vi "Diagnostic Cycle.vi"(8 "error in (no error)":errorcluster, 11 "MSX-E3711 in":refnum<class "MSX-E3711.lvclass">) -> (0 "error out":errorcluster, 3 "MSX-E3711 out":refnum<class "MSX-E3711.lvclass">)   [LabVIEW 2014, in "MSX-E3711.lvlib" / "MSX-E3711.lvclass"]
uses:
  MSX-E3711.lvclass
  MSX-E3711.lvclass/MSX-E3711.ctl
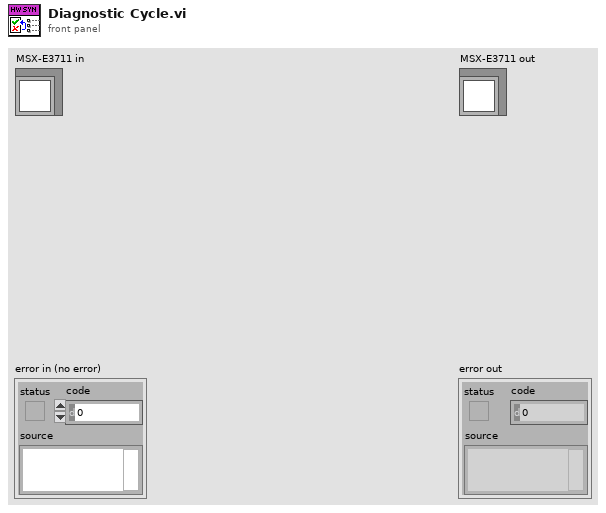
[diagram p1: front panel]
types:
  T1 = typedef "DriverMasterSync.lvlibp/WINFAS 2 Data Queue.lvlib/Acquisition Data 1 Sample Cluster.ctl" = cluster{"TDX":sgl[], "Encoder":sgl}
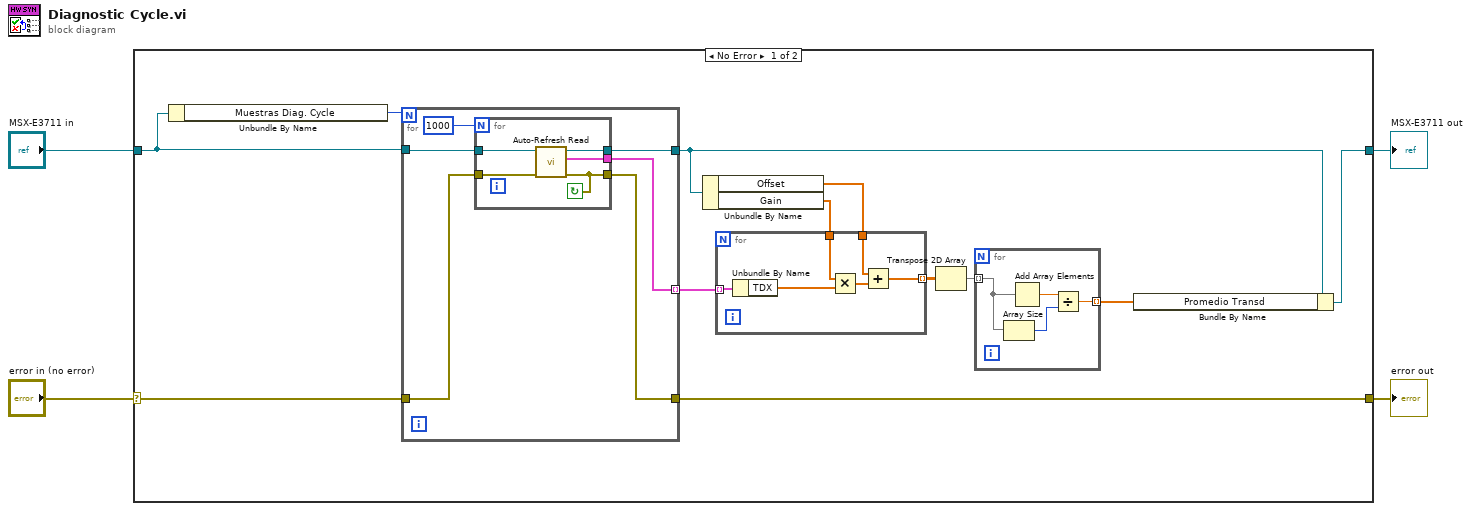
[diagram p0: block diagram]
diagram:
  n1 = case shown="No Error" "error in (no error)" {
    selector: "error in (no error)" -> [w8 w39]
    tunnel: [w5 w39] -> w3
    tunnel: [w6 w38] -> w1
    tunnel: "MSX-E3711 in" -> [w7 w38]
    frame No Error {
      n2 = Unbundle By Name(w7) -> ("Muestras Diag. Cycle"=w12:u32)
      n3 = for {
        N: w12 -> [_]
        tunnel: [w19] -> w16 mode=indexing
        tunnel: w7 -> [w17]
        tunnel: [w20] -> w11
        tunnel: w8 -> [w22]
        tunnel: [w18] -> w5
        n4 = for {
          N: 1000 -> [_]
          tunnel: w22 -> [w26]
          tunnel: w17 -> [w27]
          tunnel: [w23] -> w20
          tunnel: [w25] -> w18
          tunnel: [w24] -> w19
          stop <- w25 continue-if-true
          n5 = call-dynamic "Auto-Refresh Read.vi"("error in (no error)"=w26, "MSX-E3711 in"=w27) -> ("error out"=w25:errorcluster, "1 Sample"=w24:T1, "MSX-E3711 out"=w23:refnum<class "MSX-E3711.lvclass">)  [unwired: 6 in, 1 out]
        }
      }
      n6 = Unbundle By Name(w11) -> ("Offset"=w9:sgl[], "Gain"=w10:sgl[])
      n7 = for {
        tunnel: w16 -> [w37] mode=indexing
        tunnel: [w35] -> w14 mode=indexing
        tunnel: w10 -> [w33]
        tunnel: w9 -> [w32]
        n8 = Unbundle By Name(w37) -> ("TDX"=w34:sgl[])
        n9 = Multiply(x=w33, y=w34) -> (x*y=w36:sgl[])
        n10 = Add(x=w32, y=w36) -> (x+y=w35:sgl[])
      }
      n11 = Transpose 2D Array(2D array=w14) -> (transposed array=w13:sgl[][])
      n12 = for {
        tunnel: w13 -> [w31] mode=indexing
        tunnel: [w28] -> w15 mode=indexing
        n13 = Array Size(array=w31) -> (size(s)=w30:i32)
        n14 = Add Array Elements(numeric array=w31) -> (sum=w29:sgl)
        n15 = Divide(x=w29, y=w30) -> (x/y=w28:sgl)
      }
      n16 = Bundle By Name(cluster=w11, "Promedio Transd"=w15) -> (w6:refnum<class "MSX-E3711.lvclass">)
    }
    frame Error {
    }
  }
  "error out" <- w3
  "MSX-E3711 out" <- w1
